vi "LagDeConAllCh (SubVI).vi"(7 "new reference":refnum<k24>, 8 "error in (no error)":errorcluster, 9 "irf":dbl[][](array[numeric]), 10 "BG":dbl[][](array[numeric]), 11 "WF":dbl[][](array[numeric])) -> (0 "error out":errorcluster, 1 "LCs":dbl[][](array[numeric]), 2 "INTs":dbl[][](array[numeric]), 3 "LTs":dbl[][](array[numeric]))   [LabVIEW 2024]
uses:
  C:/Users/MarcuLab/Documents/GitHub/NetDeconForLV/Source/DotNETAssembly1.0.3/output/build/LaguerreDeconRTNative.dll
  Documents/GitHub/NetDeconForLV/Source/DotNETAssembly1.0.3/output/build/LaguerreDeconRTNative.dll
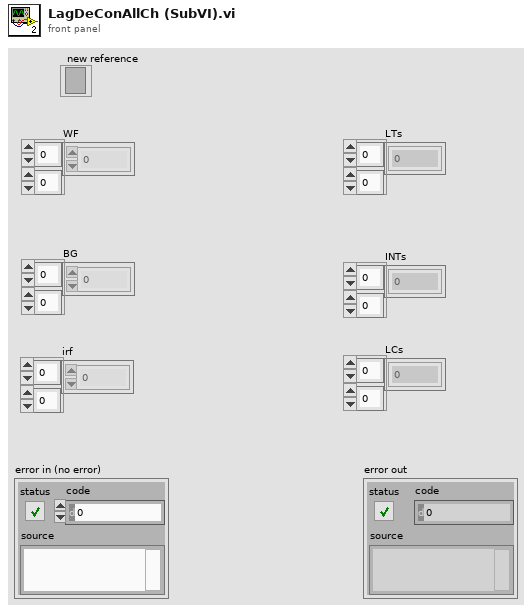
[diagram p1: front panel]
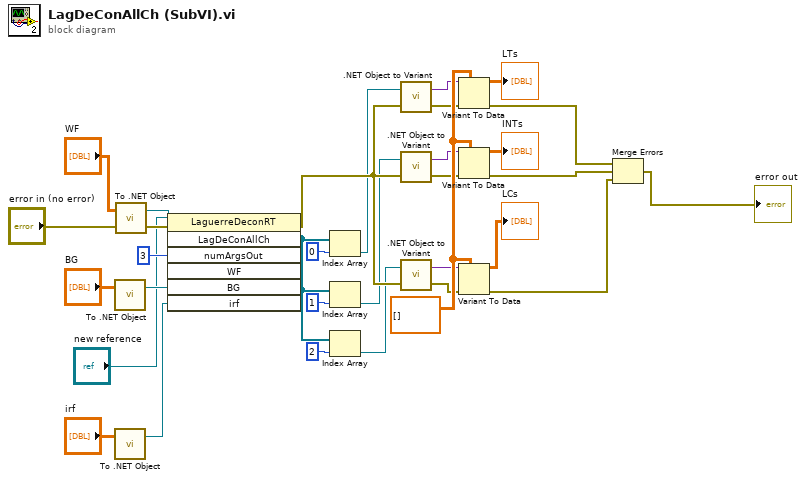
[diagram p0: block diagram]
diagram:
  w31 = dbl[][] []
  n1 = call <vilib>:"To .NET Object.vi"("anything"="BG") -> (".NET object"=w21:refnum<k24>)  [unwired: 1 in, 1 out]
  n2 = call <vilib>:"To .NET Object.vi"("anything"="irf") -> (".NET object"=w23:refnum<k24>)  [unwired: 1 in, 1 out]
  n3 = call <vilib>:"To .NET Object.vi"("error in (no error)"="error in (no error)", "anything"="WF") -> ("error out"=w10:errorcluster, ".NET object"=w11:refnum<k24>)
  n4 = invoke class="LaguerreDeconRT" method="LagDeConAllCh"(reference="new reference", error in=w10, "numArgsOut"=3, "WF"=w11, "BG"=w21, "irf"=w23) -> (error out=w28:errorcluster, "LagDeConAllCh"=w14:refnum<k24>[])  [unwired: 1 in, 5 out]
  n5 = Index Array(array=w14, index=0) -> (element=w16:refnum<k24>)
  n6 = Index Array(array=w14, index=1) -> (element=w24:refnum<k24>)
  n7 = Index Array(array=w14, index=2) -> (element=w25:refnum<k24>)
  n8 = call <vilib>:".NET Object to Variant.vi"("error in (no error)"=w28, ".NET object"=w16) -> ("error out"=w18:errorcluster, "variant"=w17:variant)
  n9 = call <vilib>:".NET Object to Variant.vi"("error in (no error)"=w28, ".NET object"=w24) -> ("error out"=w27:errorcluster, "variant"=w26:variant)
  n10 = call <vilib>:".NET Object to Variant.vi"("error in (no error)"=w28, ".NET object"=w25) -> ("error out"=w29:errorcluster, "variant"=w30:variant)
  n11 = Variant To Data(error in=w18, type=w31, Variant=w17) -> (data=→"LTs":dbl[][], error out=w4:errorcluster)
  n12 = Variant To Data(error in=w27, type=w31, Variant=w26) -> (data=→"INTs":dbl[][], error out=w3:errorcluster)
  n13 = Variant To Data(error in=w29, type=w31, Variant=w30) -> (data=→"LCs":dbl[][], error out=w2:errorcluster)
  n14 = Merge Errors(w4, w3, w2) -> (→"error out":errorcluster)
